vi "getdata.vi"(4 "Device Address":u8=2, 5 "Input Port in":T1 items=["Port 1", "Port 2", "Port 3", "Port 4"], 6 "Reg Address":u8=16, 7 "error in":errorcluster) -> (0 "Input Port out":T1 items=["Port 1", "Port 2", "Port 3", "Port 4"], 1 "data":u8[](array[numeric]), 3 "error out":errorcluster)   [LabVIEW 2016]
uses:
  <vilib>/NXT/Block Support/HWPage.SensorType.ctl
  <vilib>/NXT/Block Support/HWPage.SensorMode.ctl
  <vilib>/NXT/Block Support/NXT_InputPort.ctl
  <vilib>/NXT/Block Support/nxt.ctl
panel:
  out "size(s)":i32
  out "NXTObject dup":T2={"nxtHandle"=57958280, "fileHandle"=0, "fileIterHandle"=0, "moduleHandle"=0, "modIterHandle"=0, "nxtIterHandle"=0} {"nxtIterHandle" format="%08x"; "modIterHandle" format="%08x"; "moduleHandle" format="%08x"; "fileIterHandle" format="%08x"; "fileHandle" format="%08x"; "nxtHandle" format="%08x"}
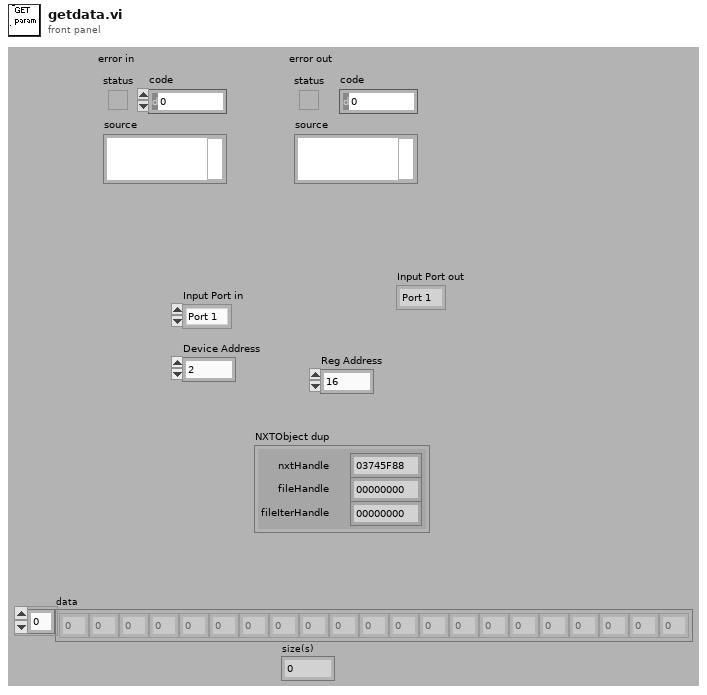
[diagram p1: front panel]
types:
  T1 = typedef "NXT_InputPort.ctl" = u32
  T2 = typedef "nxt.ctl" = cluster{"nxtHandle":u64, "fileHandle":u64, "fileIterHandle":u64, "moduleHandle":u64, "modIterHandle":u64, "nxtIterHandle":u64}
  T3 = typedef "HWPage.SensorMode.ctl" = u8
  T4 = typedef "HWPage.SensorType.ctl" = u8
  T5 = typedef "NXT_StatusCodes.ctl" = i8
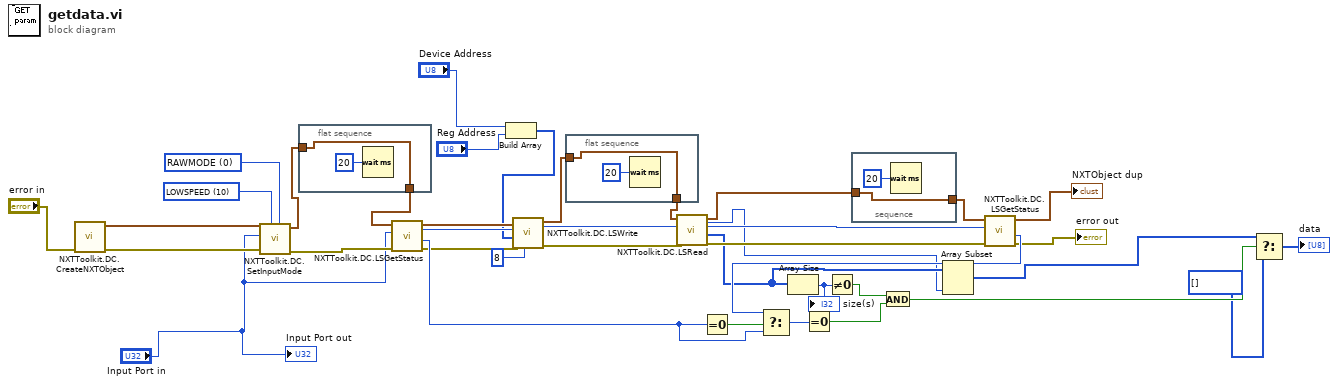
[diagram p0: block diagram]
diagram:
  w38 = T3 0 items=["RAWMODE"=0, "BOOLEANMODE"=32, "TRANSITIONCNTMODE"=64, "PERIODCOUNTERMODE"=96, "PCTFULLSCALEMODE"=128, "CELSIUSMODE"=160, "FAHRENHEITMODE"=192, "ANGLESTEPMODE"=224] ("Sensor Mode (RAWMODE)")
  w39 = T4 10 items=["NO_SENSOR", "SWITCH", "TEMPERATURE", "REFLECTION", "ANGLE", "LIGHT_ACTIVE", "LIGHT_INACTIVE", "SOUND_DB", "SOUND_DBA", "CUSTOM", "LOWSPEED", "LOWSPEED_9V", "HIGHSPEED"] ("Sensor Type (NO_SENSOR)")
  n1 = call <vilib>:"NXTToolkit.DC.CreateNXTObject.vi"("error in (no error)"="error in") -> ("error out"=w20:errorcluster, "NXTObject"=w21:T2)  [unwired: 8 in, 1 out]
  n2 = call <vilib>:"NXTToolkit.DC.SetInputMode.vi"("Sensor Mode (RAWMODE)"=w38, "Sensor Type (NO_SENSOR)"=w39, "error in (no error)"=w20, "Input Port (Port 1)"="Input Port in", "NXTObject"=w21) -> ("error out"=w37:errorcluster, "NXTObject dup"=w19:T2)  [unwired: 4 in, 1 out]
  n3 = flat-sequence {
    tunnel: w19 -> [w40]
    tunnel: [w40] -> w18
    frame #0 {
      n4 = Wait (ms)(milliseconds to wait=u32 20) -> ()  [unwired: 1 out]
    }
  }
  n5 = call <vilib>:"NXTToolkit.DC.LSGetStatus.vi"("error in (no error)"=w37, "Input Port (Port 1)"="Input Port in", "NXTObject"=w18) -> ("error out"=w29:errorcluster, "Status"=w33:T5, "Input Port dup"=w27:T1, "NXTObject dup"=w30:T2)  [unwired: 2 in, 3 out]
  n6 = Build Array("Device Address", "Reg Address") -> (w17:u8[])
  n7 = call <vilib>:"NXTToolkit.DC.LSWrite.vi"("Response Length (0)"=8, "error in (no error)"=w29, "Buffer"=w17, "Input Port (Port 1)"=w27, "NXTObject"=w30) -> ("error out"=w28:errorcluster, "Input Port dup"=w26:T1, "NXTObject dup"=w14:T2)  [unwired: 3 in, 1 out]
  n8 = flat-sequence {
    tunnel: w14 -> [w42]
    tunnel: [w42] -> w13
    frame #0 {
      n9 = Wait (ms)(milliseconds to wait=u32 20) -> ()  [unwired: 1 out]
    }
  }
  n10 = call <vilib>:"NXTToolkit.DC.LSRead.vi"("error in (no error)"=w28, "Input Port (Port 1)"=w26, "NXTObject"=w13) -> ("error out"=w31:errorcluster, "Buffer"=w3:u8[], "Input Port dup"=w25:T1, "NXTObject dup"=w32:T2, "Bytes Read"=w2:u8)  [unwired: 3 in, 1 out]
  n11 = Equal To 0?(x=w33) -> (x = 0?=w35:bool)
  n12 = Array Size(array=w3) -> (size(s)=w22:i32)
  "size(s)" <- w22
  n13 = Not Equal To 0?(x=w22) -> (x != 0?=w9:bool)
  n14 = stacked-sequence {
    tunnel: [w45] -> w36
    tunnel: w32 -> [w45]
    frame #0 {
      n15 = Wait (ms)(milliseconds to wait=u32 20) -> ()  [unwired: 1 out]
    }
  }
  n16 = Array Subset(array=w3, length=w2) -> (w1:u8[])  [unwired: 1 in]
  n17 = call <vilib>:"NXTToolkit.DC.LSGetStatus.vi"("error in (no error)"=w31, "Input Port (Port 1)"=w25, "NXTObject"=w36) -> ("error out"=→"error out":errorcluster, "Status"=w34:T5, "NXTObject dup"=→"NXTObject dup":T2)  [unwired: 2 in, 4 out]
  n18 = Select(t=w34, s=w35, f=w33) -> (s? t:f=w10:T5)
  n19 = Equal To 0?(x=w10) -> (x = 0?=w8:bool)
  n20 = And(x=w9, y=w8) -> (x .and. y?=w11:bool)
  n21 = Select(t=w1, s=w11, f=u8[] []) -> (s? t:f=→"data":u8[])
  "Input Port out" <- "Input Port in"
